vi "CPP-8116Spectra.vi"() -> (5 "Plug in titles":string[](array[string]), 7 "Plug in values":string[](array[string]))   [LabVIEW 2015]
uses:
  Globals/Meas_global.vi
panel:
  in  "Tab Control":enum32{"Graphs", "Numerics"}(tab)
  out "Spectra":T1(graph)
  out "Timetrace":dbl[][](graph)
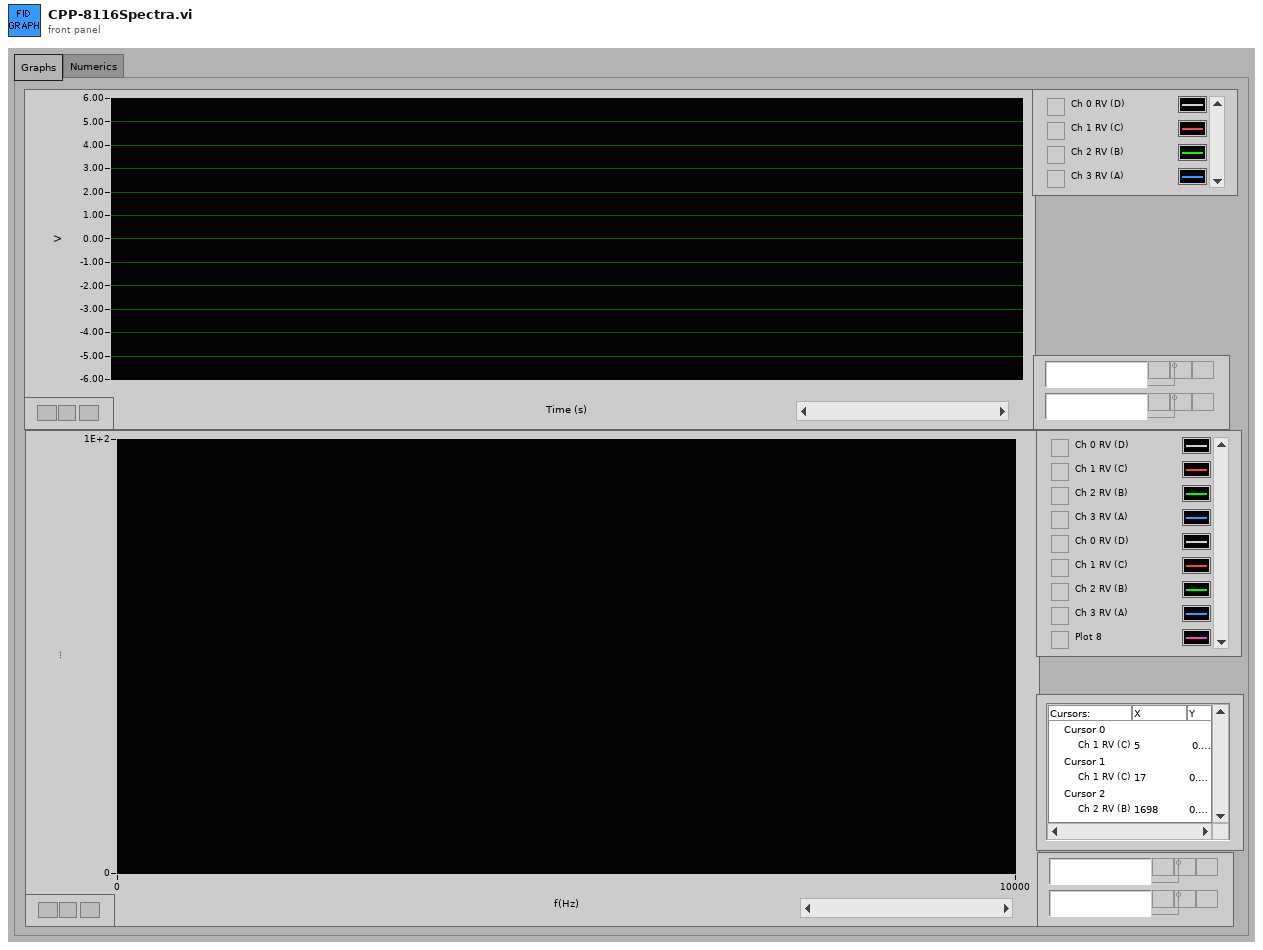
[diagram p1: front panel]
types:
  T1 = cluster{"dF":dbl, "dF":dbl, "Spectrum output array":dbl[]}[]
  T2 = typedef "Analysis_info_cluster.ctl" = cluster{"Colour":u32, "Inst type":T3, "Inst name":string, "Symbol":string, "Code name":string, "Extra Info":string, "Inst Array":T4, "Extra Titles":string[], "Extra Values":string[], "U":dbl, "u^2":dbl, "u^3":dbl, "u^4":dbl, "Skew_u":dbl, "Kurt_u":dbl, "Sd Error in Mean":dbl, "% u'/U":dbl, "X":dbl, "Y":dbl, "Z":dbl, "Timescale integral to 25%":dbl, "Sd Error in Variance":dbl, "Calib File":path, "Calib Constants":dbl[], "Output Position":bool, "Full Stats":bool, "Av Sampling Rate":dbl, "Av No of Samples":dbl, "Total Meas Time (s)":dbl, "ADAM Ch Name":string}
  T3 = typedef "Inst_type.ctl" = enum16{"Propeller anemometer", "Raw voltage", "Pressure Transducer", "Pitot-static tube", "Preston tube", "Hot wire", "Cross wire 1", "Cross wire 2", "Generic Linear", "Generic Polynomial", "Generic BackPoly", "Fast FID", "Thermocouple", "Cold wire", "Pulsed Wire", "LDA Vel", "LDA Tran time", "LDA Arr time", "Microphone"}
  T4 = typedef "Instrument_Array.ctl" = enum16{"PWA", "LDA", "Analogue"}
  T5 = typedef "Time_Trace_Cluster.ctl" = cluster{"Weighting":dbl[], "Time (s)":dbl[], "Voltage":dbl[], "Eng Values":dbl[]}
  T6 = cluster{"dF":dbl, "dF":dbl, "SingleBlockSpectrum":dbl[]}
  T7 = cluster{"dF":dbl, "dF":dbl, "SingleBlockSpectrum":dbl[]}[]
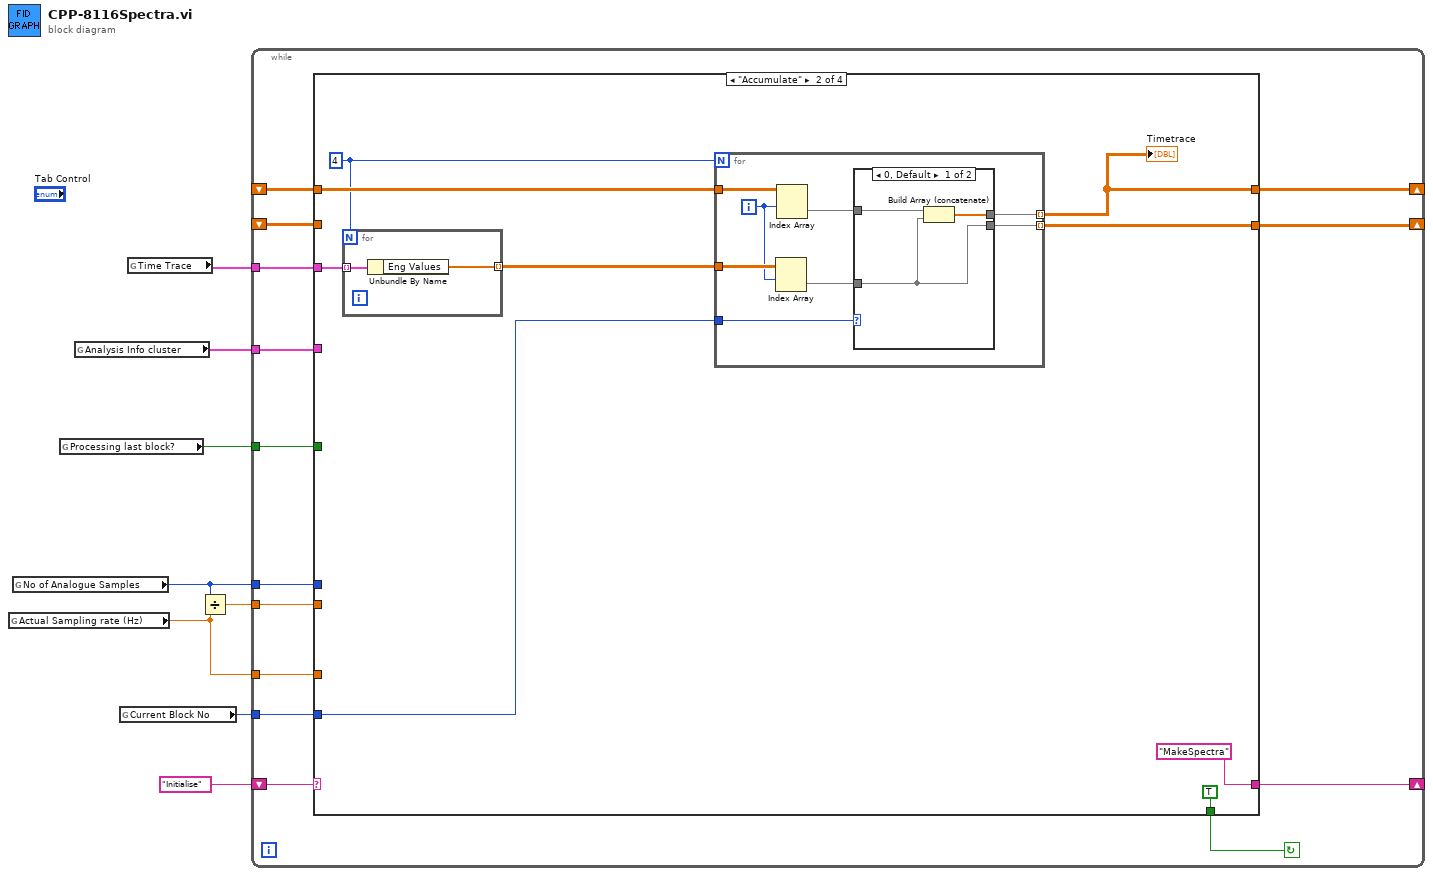
[diagram p0: block diagram]
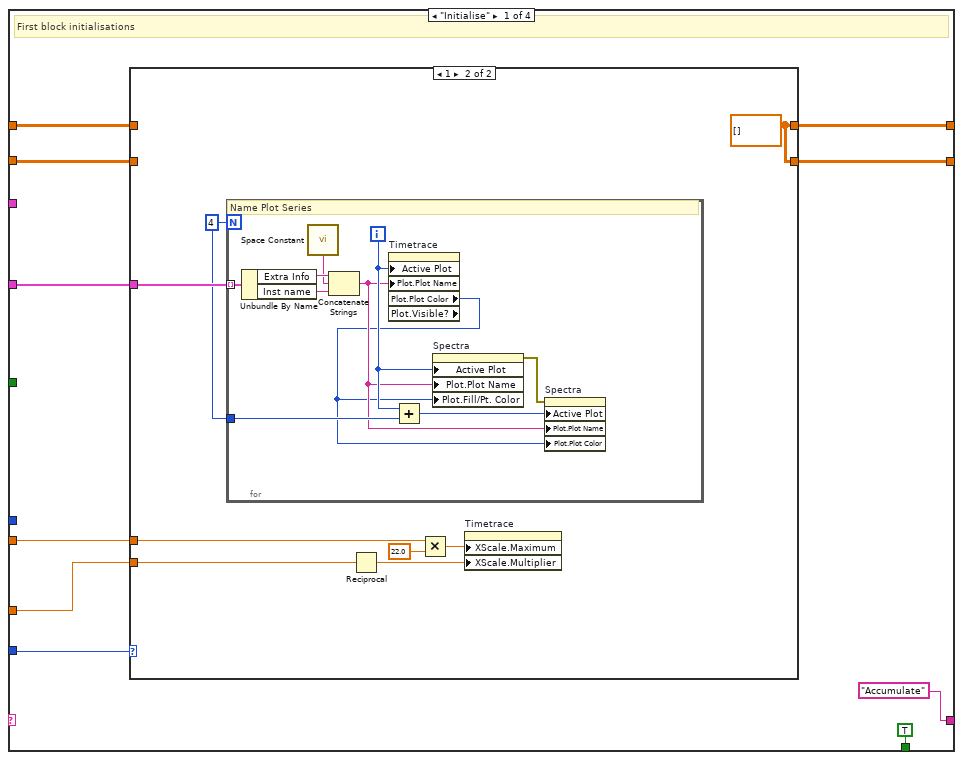
[diagram p2: hidden frame]
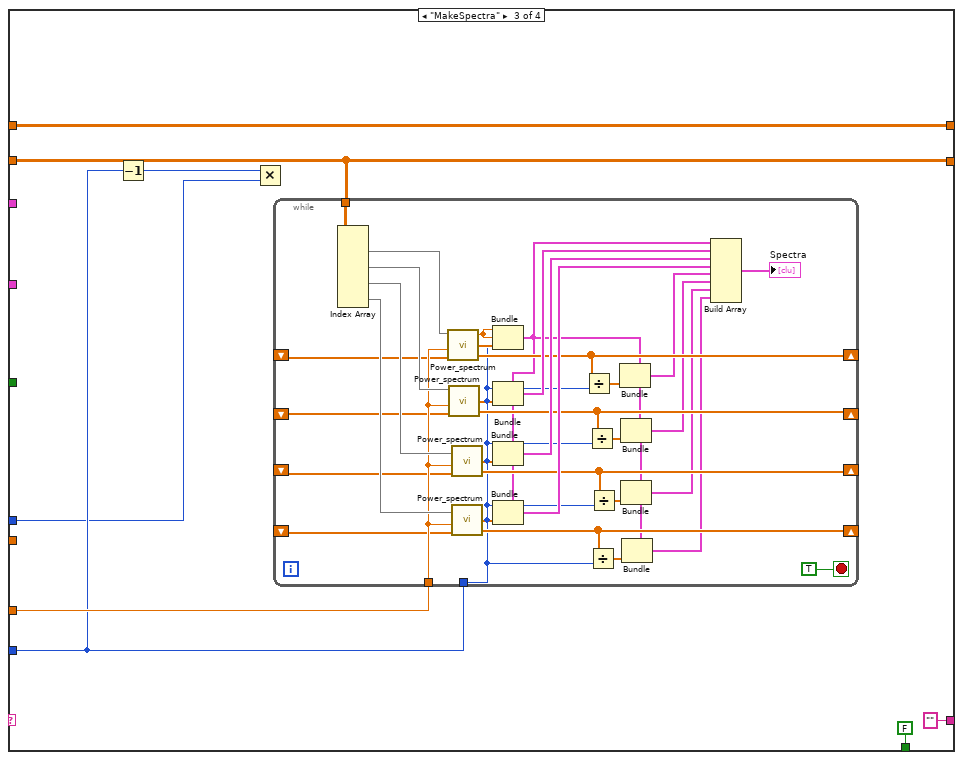
[diagram p5: hidden frame]
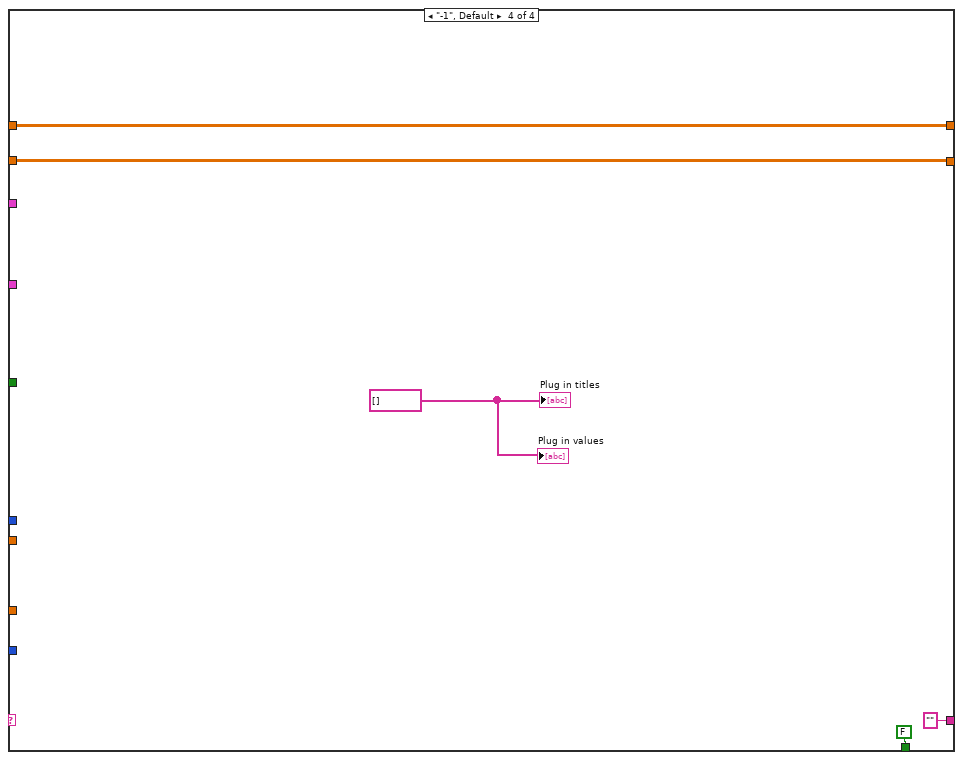
[diagram p6: hidden frame]
diagram:
  n1 = global read "Meas_global.vi" "Actual Sampling rate (Hz)"() -> (w2:dbl)
  n2 = global read "Meas_global.vi" "No of Analogue Samples"() -> (w1:i32)
  n3 = global read "Meas_global.vi" "Processing last block?"() -> (w3:bool)
  n4 = global read "Meas_global.vi" "Analysis Info cluster"() -> (w5:T2[])
  n5 = global read "Meas_global.vi" "Current Block No"() -> (w7:i32)
  n6 = global read "Meas_global.vi" "Time Trace"() -> (w8:T5[])
  n7 = Divide(x=w1, y=w2) -> (x/y=w6:dbl)
  n8 = while {
    shift-left: "Initialise" -> [w14]
    shift-right: [w20] -> _
    tunnel: w8 -> [w21]
    tunnel: w7 -> [w19]
    tunnel: w6 -> [w18]
    shift-right: [w16] -> _
    shift-left: _ -> [w17]
    tunnel: w5 -> [w15]
    tunnel: w3 -> [w13]
    tunnel: w2 -> [w12]
    tunnel: w1 -> [w11]
    shift-right: [w10] -> _
    shift-left: _ -> [w9]
    stop <- w22 continue-if-true
    n9 = case shown="\"Accumulate\"" w14 {
      tunnel: [TRUE TRUE FALSE FALSE] -> w22
      tunnel: w21 -> [_ w61 _ _]
      tunnel: ["Accumulate" "MakeSpectra" "" ""] -> w20
      tunnel: w19 -> [w27 w57 w79 _]
      tunnel: w18 -> [w31 _ _ _]
      tunnel: w15 -> [w29 _ _ _]
      tunnel: [w30 w55 w81 w121] -> w16
      tunnel: w17 -> [w26 w56 w81 w121]
      tunnel: w13 -> [_ _ _ _]
      tunnel: w12 -> [w25 _ w80 _]
      tunnel: w11 -> [_ _ w78 _]
      tunnel: [w24 w53 w76 w118] -> w10
      tunnel: w9 -> [w23 _ w76 w118]
      frame "Initialise" {
        # "First block initialisations"
        n10 = case shown="1" w27 {
          tunnel: w31 -> [_ w41]
          tunnel: [w34 w35] -> w30
          tunnel: w29 -> [_ w40]
          tunnel: w26 -> [w34 _]
          tunnel: w25 -> [_ w37]
          tunnel: [w33 w35] -> w24
          tunnel: w23 -> [w33 _]
          frame 0, Default {
          }
          frame 1 {
            w35 = dbl[][] [] ("Eng Values")
            w36 = 4
            n11 = for {
              N: w36 -> [_]
              tunnel: w40 -> [w50] mode=indexing
              tunnel: w36 -> [w47]
              i -> [w48]
              # "Name Plot Series"
              n12 = Unbundle By Name(w50) -> ("Extra Info"=w52:string, "Inst name"=w49:string)
              n13 = call <vilib>:"Space Constant.vi"() -> ("String"=w51:string)
              n14 = Concatenate Strings(w52, w51, w49) -> (w45:string)
              n15 = property on="Timetrace" class="WFGraph (strict)" props=["Active Plot", "Plot", "Plot Name", "Plot", "Plot Color", "Plot", "Visible?"]("Active Plot"=w48, "Plot.Plot Name"=w45) -> ("Plot.Plot Color"=w43:u32)  [unwired: 2 in, 3 out]
              n16 = Add(x=w48, y=w47) -> (x+y=w44:i32)
              n17 = property on="Spectra" class="WFGraph (strict)"("Active Plot"=w48, "Plot.Plot Name"=w45, "Plot.Fill/Pt. Color"=w43) -> (error out=w46:errorcluster)  [unwired: 2 in, 1 out]
              n18 = property on="Spectra" class="WFGraph (strict)"(error in=w46, "Active Plot"=w44, "Plot.Plot Name"=w45, "Plot.Plot Color"=w43) -> ()  [unwired: 1 in, 2 out]
            }
            n19 = Reciprocal(x=w37) -> (1/x=w38:dbl)
            n20 = Multiply(x=w41, y=22.0) -> (x*y=w42:dbl)
            n21 = property on="Timetrace" class="WFGraph (strict)"("XScale.Maximum"=w42, "XScale.Multiplier"=w38) -> ()  [unwired: 2 in, 2 out]
          }
        }
      }
      frame "Accumulate" {
        w54 = 4
        n22 = for {
          N: w54 -> [_]
          tunnel: w61 -> [w75] mode=indexing
          tunnel: [w74] -> w58 mode=indexing
          n23 = Unbundle By Name(w75) -> ("Eng Values"=w74:dbl[])
        }
        n24 = for {
          N: w54 -> [_]
          tunnel: w58 -> [w69]
          tunnel: [w68] -> w55 mode=indexing
          tunnel: w57 -> [w66]
          tunnel: w56 -> [w64]
          tunnel: [w62] -> w53 mode=indexing
          i -> [w63]
          n25 = Index Array(array=w69, index (row)=w63) -> (element=w65:dbl[])  [unwired: 1 in]
          n26 = Index Array(array=w64, index (row)=w63) -> (element=w67:dbl[])  [unwired: 1 in]
          n27 = case shown="0, Default" w66 {
            tunnel: w67 -> [w72 _]
            tunnel: w65 -> [w70 w73]
            tunnel: [w71 w73] -> w68
            tunnel: [w70 w73] -> w62
            frame 0, Default {
              n28 = Build Array (concatenate)(w72, w70) -> (w71:dbl[])
            }
            frame 1 {
            }
          }
        }
        "Timetrace" <- w55
      }
      frame "MakeSpectra" {
        n29 = Decrement(x=w79) -> (x-1=w77:i32)
        n30 = Multiply(x=w77, y=w78) -> ()  [unwired: 1 out]
        n31 = while {
          tunnel: w76 -> [w117]
          tunnel: w80 -> [w109]
          tunnel: w79 -> [w91]
          shift-right: [w98] -> _
          shift-left: _ -> [w104]
          shift-right: [w97] -> _
          shift-left: _ -> [w103]
          shift-right: [w96] -> _
          shift-left: _ -> [w102]
          shift-right: [w95] -> _
          shift-left: _ -> [w101]
          stop <- TRUE stop-if-true
          n32 = Index Array(array=w117) -> (element #1=w116:dbl[], element #2=w115:dbl[], element #3=w114:dbl[], element #4=w110:dbl[])  [unwired: 8 in]
          n33 = call "Power_spectrum.vi"("U"=w116, "Sampling frequency"=w109, "Spectrum input array"=w104, "Block No"=w91) -> ("dF"=w85:dbl, "SingleBlockSpectrum"=w107:dbl[], "Spectrum Accumulator array"=w98:dbl[])  [unwired: 1 in]
          n34 = call "Power_spectrum.vi"("U"=w115, "Sampling frequency"=w109, "Spectrum input array"=w103, "Block No"=w91) -> ("SingleBlockSpectrum"=w100:dbl[], "Spectrum Accumulator array"=w97:dbl[])  [unwired: 1 in, 1 out]
          n35 = call "Power_spectrum.vi"("U"=w114, "Sampling frequency"=w109, "Spectrum input array"=w102, "Block No"=w91) -> ("SingleBlockSpectrum"=w106:dbl[], "Spectrum Accumulator array"=w96:dbl[])  [unwired: 1 in, 1 out]
          n36 = call "Power_spectrum.vi"("U"=w110, "Sampling frequency"=w109, "Spectrum input array"=w101, "Block No"=w91) -> ("SingleBlockSpectrum"=w105:dbl[], "Spectrum Accumulator array"=w95:dbl[])  [unwired: 1 in, 1 out]
          n37 = Bundle("dF"=w85, "dF"=w85, "SingleBlockSpectrum"=w107) -> (w84:T6)  [unwired: 1 out]
          n38 = Bundle(cluster=w84, "SingleBlockSpectrum"=w100) -> (w113:T6)  [unwired: 2 out]
          n39 = Bundle(cluster=w84, "SingleBlockSpectrum"=w106) -> (w112:T6)  [unwired: 2 out]
          n40 = Bundle(cluster=w84, "SingleBlockSpectrum"=w105) -> (w108:T6)  [unwired: 2 out]
          n41 = Divide(x=w98, y=w91) -> (x/y=w99:dbl[])
          n42 = Divide(x=w97, y=w91) -> (x/y=w94:dbl[])
          n43 = Divide(x=w95, y=w91) -> (x/y=w92:dbl[])
          n44 = Divide(x=w96, y=w91) -> (x/y=w93:dbl[])
          n45 = Bundle(cluster=w84, "SingleBlockSpectrum"=w99) -> (w90:T6)  [unwired: 2 out]
          n46 = Bundle(cluster=w84, "SingleBlockSpectrum"=w94) -> (w89:T6)  [unwired: 2 out]
          n47 = Bundle(cluster=w84, "SingleBlockSpectrum"=w93) -> (w88:T6)  [unwired: 2 out]
          n48 = Bundle(cluster=w84, "SingleBlockSpectrum"=w92) -> (w87:T6)  [unwired: 2 out]
          n49 = Build Array(w84, w113, w112, w108, w90, w89, w88, w87) -> (→"Spectra":T7)
        }
      }
      frame "-1", Default {
        w120 = string[] [] ("Plug in titles")
        "Plug in titles" <- w120
        "Plug in values" <- w120
      }
    }
  }
